vi "DSF.Engine.Execution.Transfer.Get ID.vi"(8 "error in (no error)":errorcluster, 11 "Transfer in":refnum<class "DSF.Engine.Execution.Transfer.lvclass">) -> (0 "error out":errorcluster, 2 "id":i32, 3 "Transfer out":refnum<class "DSF.Engine.Execution.Transfer.lvclass">)   [LabVIEW 2016, in "DSF.Engine.lvlib" / "DSF.Engine.Execution.Transfer.lvclass"]
uses:
  DSF.Engine.Execution.Transfer.lvclass
  DSF.Engine.Execution.Transfer.lvclass/DSF.Engine.Execution.Transfer.ctl
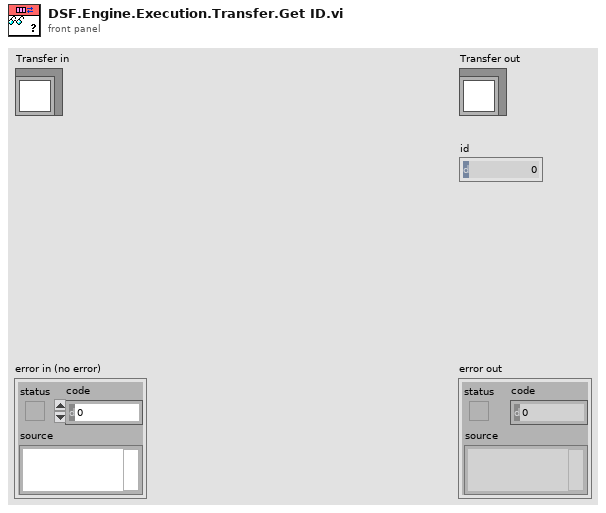
[diagram p1: front panel]
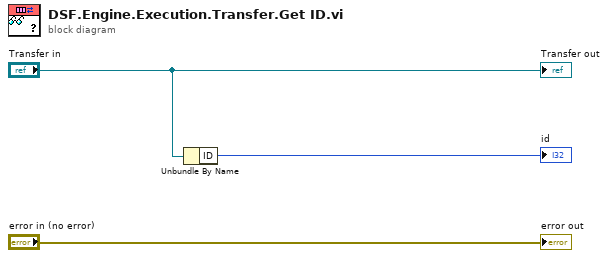
[diagram p0: block diagram]
diagram:
  n1 = Unbundle By Name("Transfer in") -> ("ID"=→"id":i32)
  "error out" <- "error in (no error)"
  "Transfer out" <- "Transfer in"
